vi "ReportListboxMean.vi"(0 "error in (no error)":errorcluster, 1 "path":path) -> (2 "error out":errorcluster, 3 "Means":string[](array[string]), 4 "Output Array":string[][](array[string]))   [LabVIEW 2013, in "main.lvlib"]
uses:
  main.lvlib
  <userlib>/_OpenG.lib/file/file.llb/File Exists - Scalar__ogtk.vi
  <vilib>/Utility/file.llb/Read From Spreadsheet File (DBL).vi
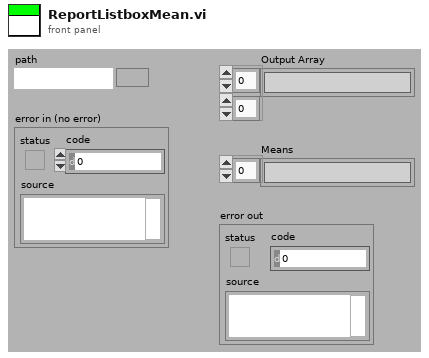
[diagram p1: front panel]
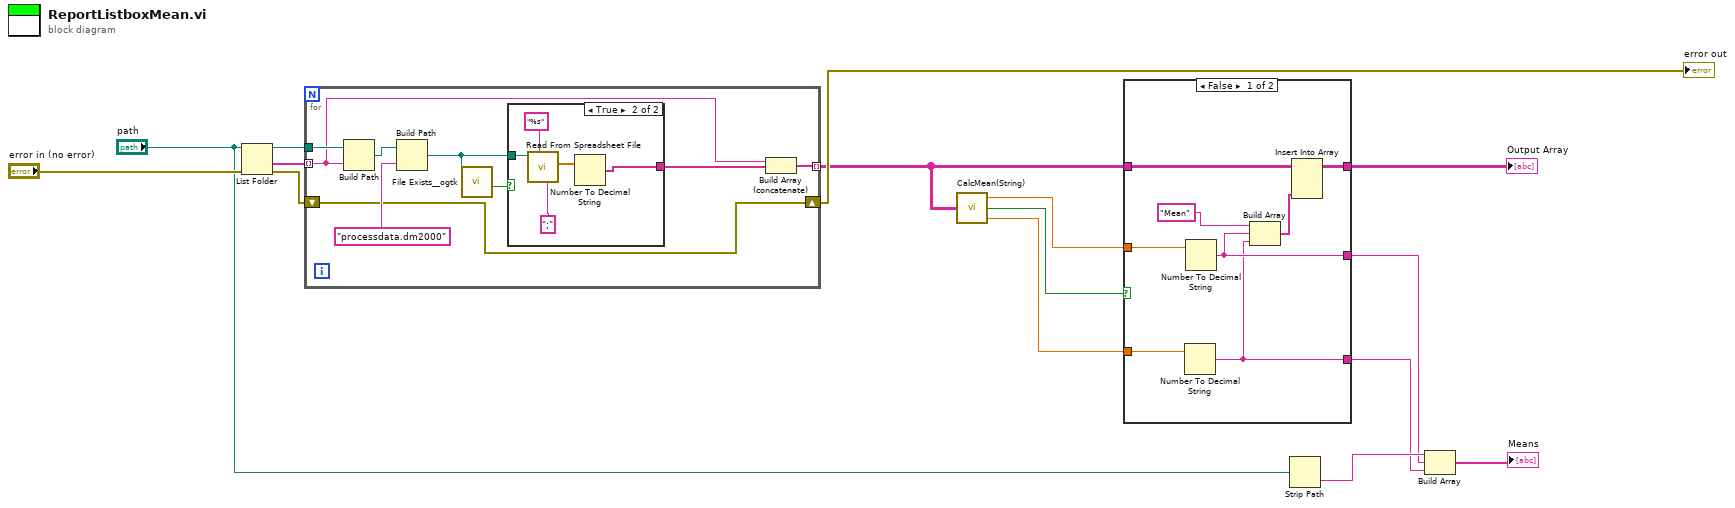
[diagram p0: block diagram]
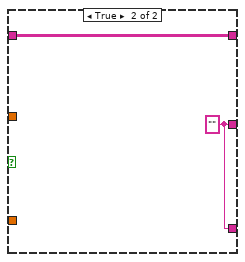
[diagram p2: hidden frame]
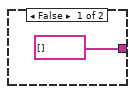
[diagram p3: hidden frame]
diagram:
  n1 = List Folder(path="path", error in="error in (no error)") -> (path out=w8:path, folder names=w7:string[], error out=w12:errorcluster)  [unwired: 2 in, 1 out]
  n2 = for {
    tunnel: w8 -> [w23]
    tunnel: w7 -> [w20] mode=indexing
    tunnel: [w19] -> w6 mode=indexing
    shift-right: [w16] -> w13
    shift-left: w12 -> [w16]
    n3 = Build Path(base path=w23, name or relative path=w20) -> (appended path=w22:path)
    n4 = Build Path(base path=w22, name or relative path="processdata.dm2000") -> (appended path=w17:path)
    n5 = call-poly <userlib>:"File Exists__ogtk.vi"("file path"=w17) -> ("exists"=w18:bool)  [unwired: 6 in, 1 out]
    n6 = case shown="True" w18 {
      tunnel: w17 -> [_ w29]
      tunnel: [string[] [] w26] -> w21
      frame False {
      }
      frame True {
        n7 = call-poly <vilib>:"Read From Spreadsheet File.vi"("delimiter (\\t)"=";" ("delimiter (\\t)"), "format (%.3f)"="%s", "file path (dialog if empty)"=w29) -> ("first row"=w27:dbl[])  [unwired: 4 in, 4 out]
        n8 = Number To Decimal String(number=w27) -> (decimal integer string=w26:string[])  [unwired: 1 in]
      }
    }
    n9 = Build Array (concatenate)(w20, w21) -> (w19:string[])
  }
  "error out" <- w13
  n10 = call "CalcMean(String).vi"("Array"=w6) -> ("Red"=w15:dbl, "Zero?"=w9:bool, "Blue"=w14:dbl)
  n11 = case shown="False" w9 {
    tunnel: w6 -> [w38 w40]
    tunnel: [w36 w40] -> w11
    tunnel: w14 -> [w35 _]
    tunnel: w15 -> [w34 _]
    tunnel: [w32 w39] -> w3
    tunnel: [w31 w39] -> w2
    frame False {
      n12 = Number To Decimal String(number=w34) -> (decimal integer string=w31:string)  [unwired: 1 in]
      n13 = Number To Decimal String(number=w35) -> (decimal integer string=w32:string)  [unwired: 1 in]
      n14 = Build Array("Mean", w32, w31) -> (w33:string[])
      n15 = Insert Into Array(array=w38, new element=w33) -> (w36:string[][])  [unwired: 2 in]
    }
    frame True {
      w39 = ""
    }
  }
  "Output Array" <- w11
  n16 = Strip Path(path="path") -> (name=w4:string)  [unwired: 1 out]
  n17 = Build Array(w4, w3, w2) -> (→"Means":string[])
